vi "Incoming Messages.vi"(8 "error in (no error)":errorcluster, 11 "Node Ptr":T3 format="%.0x") -> (0 "error out":errorcluster)   [LabVIEW 2009, in "NI-XNET Custom Device.lvlib"]
uses:
  NI-XNET Custom Device.lvlib
  <vilib>/NI VeriStand/Custom Device API/Custom Device Item Ref.ctl
  Add Selected.ctl
  Add All.ctl
  <vilib>/xnet/xnet.llb/XNET String To IO Name (Cluster).vi
  <vilib>/NI VeriStand/Custom Device API/Get Item Property (String).vi
  <vilib>/NI VeriStand/Custom Device API/Set Item Property (Variant).vi
  <vilib>/NI VeriStand/Custom Device API/Custom Device API.lvlib
  Program Files/National Instruments/LabVIEW 2009/resource/objmgr/xnet.rc
panel:
  out "Channel Assignments":u32[](array[numeric])
  out "Identifiers":u32[](array[numeric])
  out "In Cycle Repetitions?":bool
  out "Cycle Repetition":u32
  out "Channel Assignment":u32(ring)=1 items=["A"=1, "B"=2, "A and B"=3]
  out "Preamble":bool
  out "Startup":bool
  out "Sync":bool
  in  "Header 4":cluster{"Section Name 2":string}={"Section Name 2"="FlexRay Specific Settings"}
  in  "Add All":T1
  in  "Header 3":cluster{"Section Name 2":string}={"Section Name 2"="Frame Timing"}
  in  "Header 2":cluster{"Section Name 2":string}={"Section Name 2"="Frame Settings"}
  out "Default Payload":u8[](array[numeric])
  out "Transmit Time":dbl
  out "Timing Type":u32(ring) items=["Cyclic Data", "Event Data", "Cyclic Remote", "Event Remote"]
  out "Extended Identifier?":bool
  out "Payload Length":u32
  out "Identifier":u32
  in  "Add Frame":T2
  in  "Frame Selection":i32(listbox)
  in  "Header":cluster{"Section Name 2":string}={"Section Name 2"="Frame Selection"}
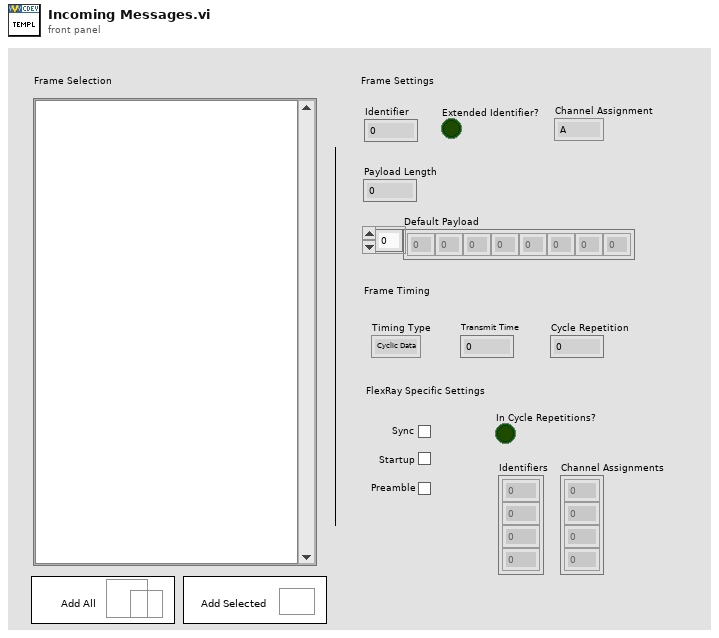
[diagram p1: front panel]
types:
  T1 = typedef "NI-XNET Custom Device.lvlib/Add All.ctl" = bool
  T2 = typedef "NI-XNET Custom Device.lvlib/Add Selected.ctl" = bool
  T3 = typedef "Custom Device API.lvlib/Custom Device Item Ref.ctl" = u64
  T4 = typedef "Custom Device API.lvlib/Custom Device Commands.ctl" = enum16{"Default", "Item renamed", "Shutdown"}
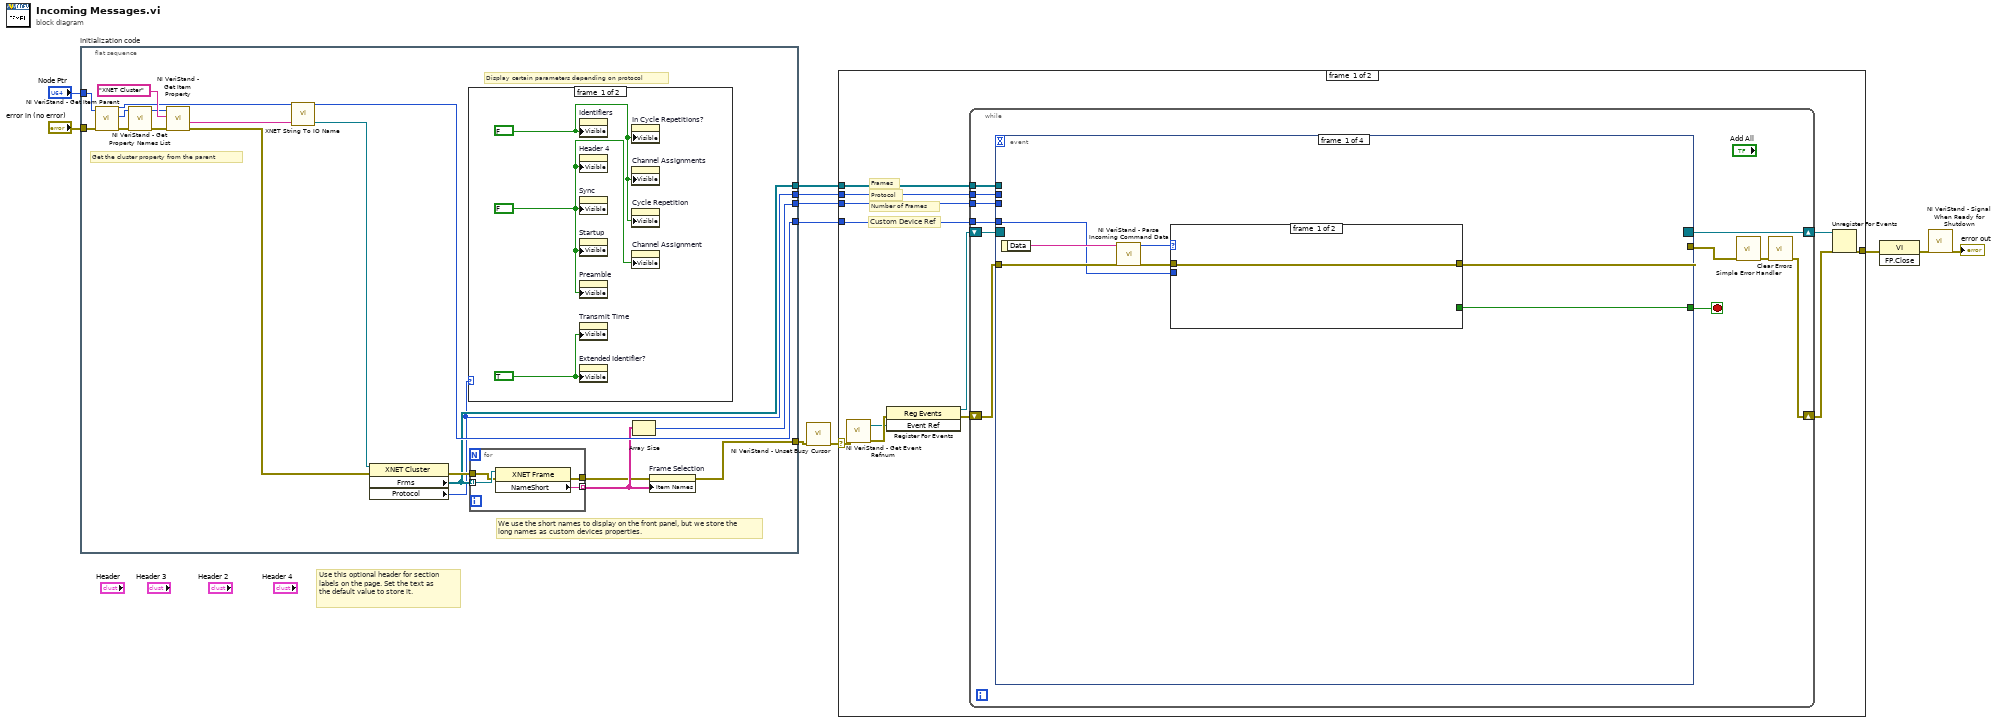
[diagram p0: block diagram]
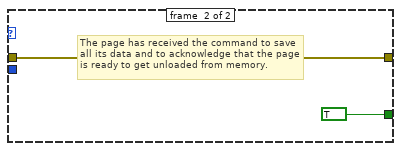
[diagram p2: hidden frame]
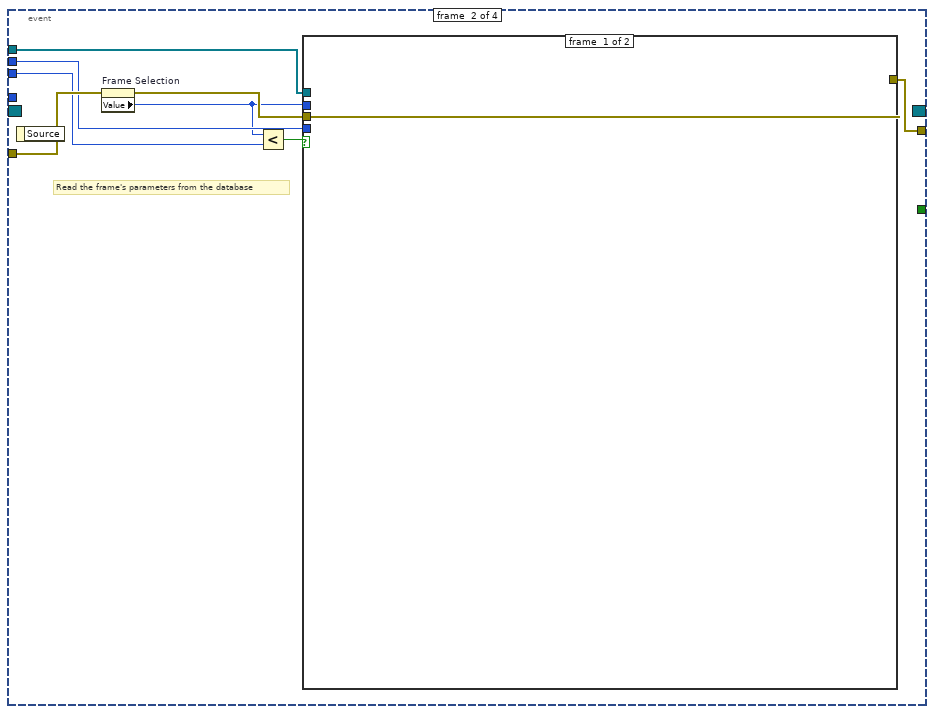
[diagram p3: hidden frame]
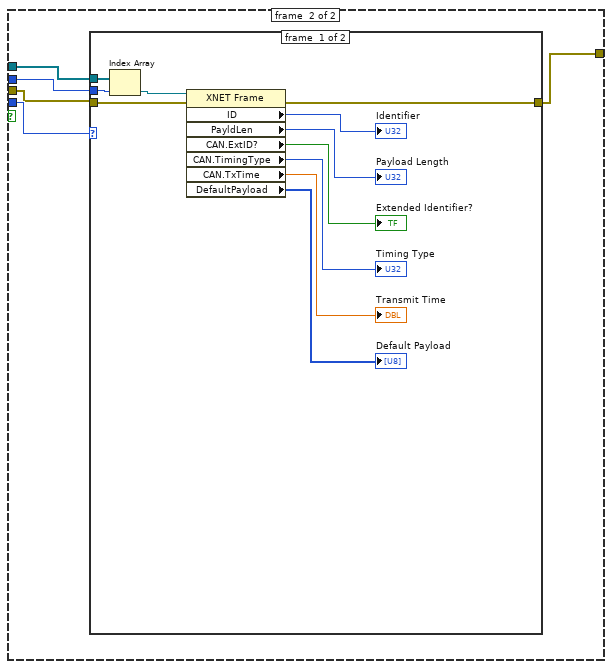
[diagram p4: hidden frame]
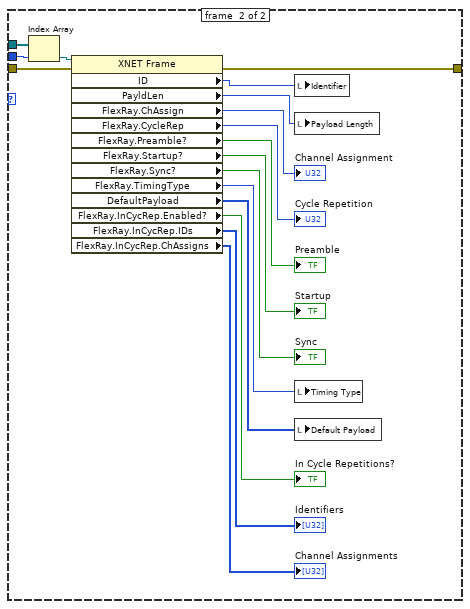
[diagram p5: hidden frame]
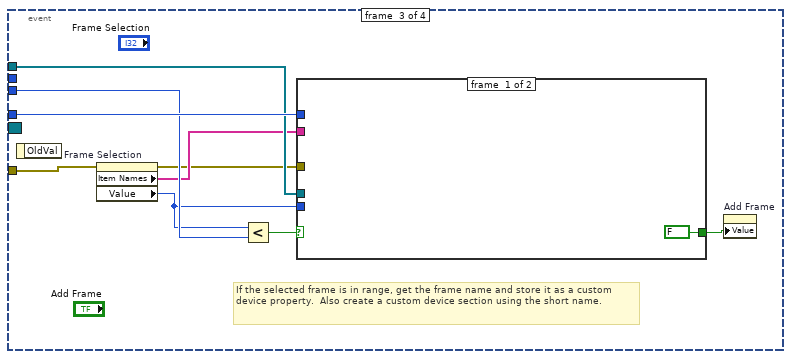
[diagram p6: hidden frame]
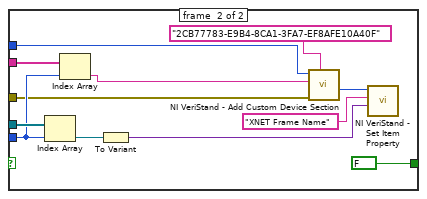
[diagram p7: hidden frame]
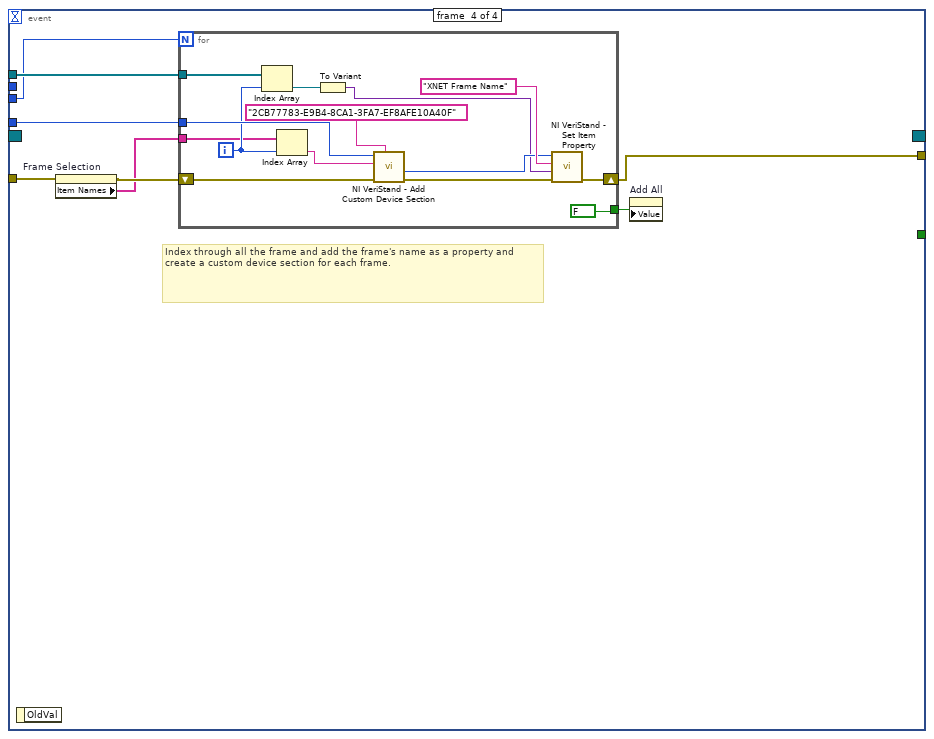
[diagram p8: hidden frame]
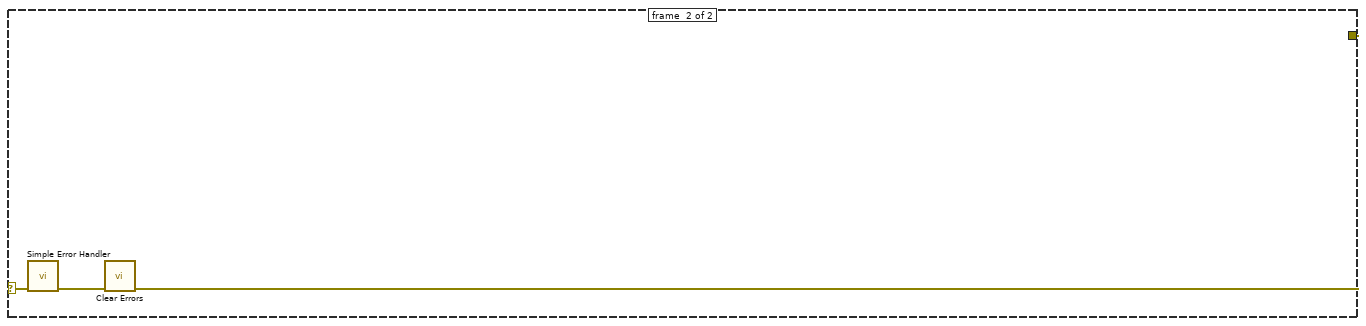
[diagram p9: hidden frame]
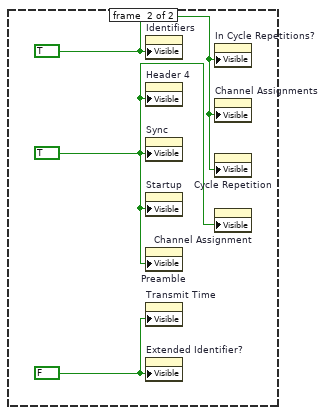
[diagram p10: hidden frame]
diagram:
  # "Use this optional header for section labels on the page. Set the text as the default value to store it."
  n1 = flat-sequence "Initialization code" {
    tunnel: "error in (no error)" -> [w16]
    tunnel: "Node Ptr" -> [w17]
    tunnel: [w12] -> w8
    tunnel: [w27] -> w5
    tunnel: [w19] -> w3
    tunnel: [w18] -> w2
    tunnel: [w15] -> w1
    frame #0 {
      # "We use the short names to display on the front panel, but we store the \nlong names as custom devices properties."
      # "Display certain parameters depending on protocol"
      # "Get the cluster property from the parent"
      n2 = call <vilib>:"NI VeriStand - Get Item Parent.vi"("error in (no error)"=w16, "Parent Ref in"=w17) -> ("error out"=w26:errorcluster, "Parent Ref"=w28:T3, "Parent Ref out"=w27:T3)  [unwired: 6 in, 1 out]
      n3 = call <vilib>:"NI VeriStand - Get Property Names List.vi"("error in (no error)"=w26, "Item Ref in"=w28) -> ("error out"=w24:errorcluster, "Item Ref out"=w25:T3)  [unwired: 7 in, 1 out]
      n4 = call-poly <vilib>:"NI VeriStand - Get Item Property.vi"("error in (no error)"=w24, "Property Name"="XNET Cluster", "Item Ref in"=w25) -> ("error out"=w22:errorcluster, "Value"=w20:string)  [unwired: 5 in, 2 out]
      n5 = call-poly <vilib>:"XNET String To IO Name.vi"("string"=w20) -> ("XNET Cluster"=w23:refnum<k21>)  [unwired: 4 in]
      n6 = property class="XNET Cluster"(reference=w23, error in=w22) -> (error out=w21:errorcluster, "Frms"=w19:refnum<k21>[], "Protocol"=w15:u32)  [unwired: 1 out]
      n7 = case shown="0, Default" w15 {
        frame #0 {
          w30 = FALSE ("Visible")
          w31 = FALSE ("Visible")
          w32 = TRUE ("Visible")
          n8 = property on="Identifiers" class="Arr (strict)"("Visible"=w30) -> ()  [unwired: 2 in, 2 out]
          n9 = property on="Header 4" class="Clust (strict)"("Visible"=w31) -> ()  [unwired: 2 in, 2 out]
          n10 = property on="Sync" class="Bool (strict)"("Visible"=w31) -> ()  [unwired: 2 in, 2 out]
          n11 = property on="Startup" class="Bool (strict)"("Visible"=w31) -> ()  [unwired: 2 in, 2 out]
          n12 = property on="Preamble" class="Bool (strict)"("Visible"=w31) -> ()  [unwired: 2 in, 2 out]
          n13 = property on="Transmit Time" class="DigNum (strict)"("Visible"=w32) -> ()  [unwired: 2 in, 2 out]
          n14 = property on="Extended Identifier?" class="Bool (strict)"("Visible"=w32) -> ()  [unwired: 2 in, 2 out]
          n15 = property on="In Cycle Repetitions?" class="Bool (strict)"("Visible"=w30) -> ()  [unwired: 2 in, 2 out]
          n16 = property on="Channel Assignments" class="Arr (strict)"("Visible"=w30) -> ()  [unwired: 2 in, 2 out]
          n17 = property on="Cycle Repetition" class="DigNum (strict)"("Visible"=w30) -> ()  [unwired: 2 in, 2 out]
          n18 = property on="Channel Assignment" class="Ring (strict)"("Visible"=w31) -> ()  [unwired: 2 in, 2 out]
        }
        frame #1 {
          w33 = TRUE ("Visible")
          w34 = TRUE ("Visible")
          w35 = FALSE ("Visible")
          n19 = property on="Identifiers" class="Arr (strict)"("Visible"=w33) -> ()  [unwired: 2 in, 2 out]
          n20 = property on="Header 4" class="Clust (strict)"("Visible"=w34) -> ()  [unwired: 2 in, 2 out]
          n21 = property on="Sync" class="Bool (strict)"("Visible"=w34) -> ()  [unwired: 2 in, 2 out]
          n22 = property on="Startup" class="Bool (strict)"("Visible"=w34) -> ()  [unwired: 2 in, 2 out]
          n23 = property on="Preamble" class="Bool (strict)"("Visible"=w34) -> ()  [unwired: 2 in, 2 out]
          n24 = property on="Transmit Time" class="DigNum (strict)"("Visible"=w35) -> ()  [unwired: 2 in, 2 out]
          n25 = property on="Extended Identifier?" class="Bool (strict)"("Visible"=w35) -> ()  [unwired: 2 in, 2 out]
          n26 = property on="In Cycle Repetitions?" class="Bool (strict)"("Visible"=w33) -> ()  [unwired: 2 in, 2 out]
          n27 = property on="Channel Assignments" class="Arr (strict)"("Visible"=w33) -> ()  [unwired: 2 in, 2 out]
          n28 = property on="Cycle Repetition" class="DigNum (strict)"("Visible"=w33) -> ()  [unwired: 2 in, 2 out]
          n29 = property on="Channel Assignment" class="Ring (strict)"("Visible"=w34) -> ()  [unwired: 2 in, 2 out]
        }
      }
      n30 = for {
        tunnel: w19 -> [w39] mode=indexing
        tunnel: [w38] -> w14 mode=indexing
        tunnel: w21 -> [w37]
        tunnel: [w36] -> w13
        n31 = property class="XNET Frame"(reference=w39, error in=w37) -> (error out=w36:errorcluster, "NameShort"=w38:string)  [unwired: 1 out]
      }
      n32 = Array Size(array=w14) -> (size(s)=w18:i32)
      n33 = property on="Frame Selection" class="LstBox (strict)"(error in=w13, "Item Names"=w14) -> (error out=w12:errorcluster)  [unwired: 1 in, 1 out]
    }
  }
  n34 = call <vilib>:"NI VeriStand - Unset Busy Cursor.vi"("error in (no error)"=w8) -> ("error out"=w7:errorcluster)  [unwired: 10 out]
  n35 = case shown="No Error" w7 {
    selector: w7 -> [w43 w161]
    tunnel: [w48 w159] -> w11
    tunnel: w5 -> [w44 _]
    tunnel: w3 -> [w42 _]
    tunnel: w2 -> [w41 _]
    tunnel: w1 -> [w40 _]
    frame #0 {
      # "Custom Device Ref"
      # "Number of Frames"
      # "Protocol"
      # "Frames"
      n36 = call <vilib>:"NI VeriStand - Get Event Refnum.vi"("error in (no error)"=w43) -> ("error out"=w51:errorcluster, "Event Ref"=w47:refnum<user-event>)  [unwired: 9 out]
      n37 = register-events(error in=w51, w47) -> (reference out=w45:refnum<event-registration>, error out=w46:errorcluster)  [unwired: 1 in]
      n38 = while {
        tunnel: w44 -> [w55]
        shift-right: [w57] -> w49
        shift-left: w46 -> [w61]
        shift-right: [w62] -> w50
        shift-left: w45 -> [w60]
        tunnel: w42 -> [w54]
        tunnel: w41 -> [w53]
        tunnel: w40 -> [w52]
        stop <- w56 stop-if-true
        n39 = event shown="[3] \"Add All\": Value Change" {
          selector: w60 -> [_ _ _ _]
          dyn-events: [_ _ _ _] -> w62
          timeout: _ -> [_ _ _ _]
          tunnel: w61 -> [w69 w79 w119 w139]
          tunnel: [w65 _ _ _] -> w56
          tunnel: [w64 w74 _ w141] -> w59
          tunnel: w55 -> [w63 _ w123 w144]
          tunnel: w54 -> [_ w80 w122 w143]
          tunnel: w53 -> [_ w78 w121 w142]
          tunnel: w52 -> [_ w76 _ _]
          event #0 {
            n40 = event-data() -> ("Data"=w68:string)  [unwired: 1 out]
            n41 = call <vilib>:"NI VeriStand - Parse Incoming Command Data.vi"("error in (no error)"=w69, "Data"=w68) -> ("error out"=w67:errorcluster, "Action"=w66:T4)  [unwired: 8 out]
            n42 = case shown="\"Shutdown\"" w66 {
              tunnel: w67 -> [w70 w71]
              tunnel: [_ TRUE] -> w65
              tunnel: [w70 w71] -> w64
              tunnel: w63 -> [_ _]
              frame #0 {
              }
              frame #1 {
                # "The page has received the command to save all its data and to acknowledge that the page is ready to get unloaded from memory."
              }
            }
          }
          event #1 {
            # "Read the frame's parameters from the database"
            n43 = event-data() -> ()  [unwired: 2 out]
            n44 = property on="Frame Selection" class="LstBox (strict)"(error in=w79) -> (error out=w75:errorcluster, "Value"=w73:i32)  [unwired: 1 in, 1 out]
            n45 = Less?(x=w73, y=w78) -> (x < y?=w77:bool)
            n46 = case shown="True" w77 {
              tunnel: w80 -> [_ w86]
              tunnel: w73 -> [_ w85]
              tunnel: w76 -> [_ w84]
              tunnel: w75 -> [w81 w83]
              tunnel: [w81 w82] -> w74
              frame #0 {
              }
              frame #1 {
                n47 = case shown="1" w84 {
                  tunnel: w86 -> [w97 w113]
                  tunnel: w85 -> [w89 w112]
                  tunnel: w83 -> [w88 w114]
                  tunnel: [w87 w110] -> w82
                  frame #0 {
                    n48 = Index Array(array=w97, index=w89) -> (element=w96:refnum<k21>)
                    n49 = property class="XNET Frame"(reference=w96, error in=w88) -> (error out=w87:errorcluster, "ID"=→"Identifier":u32, "PayldLen"=→"Payload Length":u32, "CAN.ExtID?"=→"Extended Identifier?":bool, "CAN.TimingType"=→"Timing Type":u32, "CAN.TxTime"=→"Transmit Time":dbl, "DefaultPayload"=→"Default Payload":u8[])  [unwired: 1 out]
                  }
                  frame #1 {
                    n50 = Index Array(array=w113, index=w112) -> (element=w111:refnum<k21>)
                    n51 = property class="XNET Frame"(reference=w111, error in=w114) -> (error out=w110:errorcluster, "ID"=w109:u32, "PayldLen"=w108:u32, "FlexRay.ChAssign"=→"Channel Assignment":u32, "FlexRay.CycleRep"=→"Cycle Repetition":u32, "FlexRay.Preamble?"=→"Preamble":bool, "FlexRay.Startup?"=→"Startup":bool, "FlexRay.Sync?"=→"Sync":bool, "FlexRay.TimingType"=w102:u32, "DefaultPayload"=w101:u8[], "FlexRay.InCycRep.Enabled?"=→"In Cycle Repetitions?":bool, "FlexRay.InCycRep.IDs"=→"Identifiers":u32[], "FlexRay.InCycRep.ChAssigns"=→"Channel Assignments":u32[])  [unwired: 1 out]
                    n52 = local write "Identifier"(w109) -> ()
                    n53 = local write "Payload Length"(w108) -> ()
                    n54 = local write "Timing Type"(w102) -> ()
                    n55 = local write "Default Payload"(w101) -> ()
                  }
                }
              }
            }
          }
          event #2 {
            # "If the selected frame is in range, get the frame name and store it as a custom device property.  Also create a custom device section using the short name."
            n56 = event-data() -> ()  [unwired: 2 out]
            n57 = property on="Frame Selection" class="LstBox (strict)"(error in=w119) -> (error out=w115:errorcluster, "Item Names"=w116:string[], "Value"=w117:i32)  [unwired: 1 in, 1 out]
            n58 = Less?(x=w117, y=w121) -> (x < y?=w120:bool)
            n59 = case shown="True" w120 {
              tunnel: w123 -> [_ w136]
              tunnel: w122 -> [_ w135]
              tunnel: [FALSE FALSE] -> w118
              tunnel: w117 -> [_ w128]
              tunnel: w116 -> [_ w127]
              tunnel: w115 -> [_ w126]
              frame #0 {
              }
              frame #1 {
                n60 = Index Array(array=w135, index=w128) -> (element=w130:refnum<k21>)
                n61 = Index Array(array=w127, index=w128) -> (element=w125:string)
                n62 = To Variant(anything=w130) -> (Variant=w131:variant)
                n63 = call <vilib>:"NI VeriStand - Add Custom Device Section.vi"("GUID (Default Section)"="2CB77783-E9B4-8CA1-3FA7-EF8AFE10A40F", "error in (no error)"=w126, "Section Name"=w125, "Parent Ref in"=w136) -> ("Section Ptr"=w132:T3)  [unwired: 5 in, 2 out]
                n64 = call-poly <vilib>:"NI VeriStand - Set Item Property.vi"("Value"=w131, "Property Name"="XNET Frame Name", "Item Ref in"=w132) -> ()  [unwired: 6 in, 3 out]
              }
            }
            n65 = property on="Add Frame" class="Bool (strict)"("Value"=w118) -> ()  [unwired: 2 in, 2 out]
          }
          event #3 {
            # "Index through all the frame and add the frame's name as a property and create a custom device section for each frame."
            n66 = event-data() -> ()  [unwired: 2 out]
            n67 = property on="Frame Selection" class="LstBox (strict)"(error in=w139) -> (error out=w138:errorcluster, "Item Names"=w137:string[])  [unwired: 1 in, 1 out]
            n68 = for {
              N: w142 -> [_]
              tunnel: w144 -> [w158]
              tunnel: w143 -> [w152]
              shift-right: [w149] -> w141
              shift-left: w138 -> [w148]
              tunnel: [FALSE] -> w140
              tunnel: w137 -> [w146]
              i -> [w151]
              n69 = Index Array(array=w152, index=w151) -> (element=w153:refnum<k21>)
              n70 = Index Array(array=w146, index=w151) -> (element=w145:string)
              n71 = To Variant(anything=w153) -> (Variant=w154:variant)
              n72 = call <vilib>:"NI VeriStand - Add Custom Device Section.vi"("GUID (Default Section)"="2CB77783-E9B4-8CA1-3FA7-EF8AFE10A40F", "error in (no error)"=w148, "Section Name"=w145, "Parent Ref in"=w158) -> ("error out"=w150:errorcluster, "Section Ptr"=w155:T3)  [unwired: 5 in, 1 out]
              n73 = call-poly <vilib>:"NI VeriStand - Set Item Property.vi"("error in (no error)"=w150, "Value"=w154, "Property Name"="XNET Frame Name", "Item Ref in"=w155) -> ("error out"=w149:errorcluster)  [unwired: 5 in, 2 out]
            }
            n74 = property on="Add All" class="Bool (strict)"("Value"=w140) -> ()  [unwired: 2 in, 2 out]
          }
        }
        n75 = call <vilib>:"Simple Error Handler.vi"("error in (no error)"=w59) -> ("error out"=w58:errorcluster)  [unwired: 1 in, 7 out]
        n76 = call <vilib>:"Clear Errors.vi"("error in (no error)"=w58) -> ("error out"=w57:errorcluster)  [unwired: 6 out]
      }
      n77 = Unregister For Events(event registration refnum=w50, error in=w49) -> (error out=w48:errorcluster)
    }
    frame #1 {
      n78 = call <vilib>:"Simple Error Handler.vi"("error in (no error)"=w161) -> ("error out"=w160:errorcluster)  [unwired: 1 in, 7 out]
      n79 = call <vilib>:"Clear Errors.vi"("error in (no error)"=w160) -> ("error out"=w159:errorcluster)  [unwired: 6 out]
    }
  }
  n80 = invoke class="VI" method="FP.Close"(error in=w11) -> (error out=w10:errorcluster)  [unwired: 2 in, 2 out]
  n81 = call <vilib>:"NI VeriStand - Signal When Ready for Shutdown.vi"("error in (no error)"=w10) -> ("error out"=→"error out":errorcluster)  [unwired: 10 out]
